vi "MG3700 Reset.vi"(0 "VISA In":refnum<visa-resource-name>, 1 "Error in (no error)":errorcluster) -> (2 "VISA Out":refnum<visa-resource-name>, 3 "Error code":i32, 4 "Error out":errorcluster)   [LabVIEW 2015]
doc: "Function: Resets a device to a level 3 state."
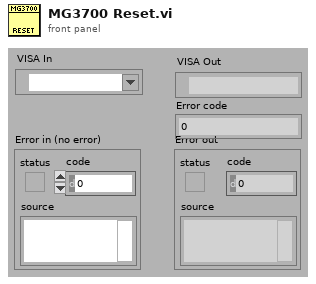
[diagram p1: front panel]
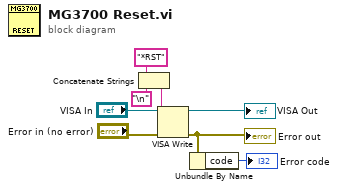
[diagram p0: block diagram]
diagram:
  n1 = Concatenate Strings("*RST" ("_Command"), "\n") -> (w2:string)
  n2 = VISA Write(VISA resource name="VISA In", write buffer=w2, error in (no error)="Error in (no error)") -> (VISA resource name out=→"VISA Out":refnum<visa-resource-name>, error out=w6:errorcluster)  [unwired: 1 out]
  "Error out" <- w6
  n3 = Unbundle By Name(w6) -> ("code"=→"Error code":i32)
